vi "Get Next.vi"(7 "Q Ref In":refnum<queue>, 8 "error in":errorcluster) -> (0 "error out":errorcluster, 2 "Packet ID":string, 3 "Payload":variant, 5 "Q Ref Out":refnum<queue>)   [LabVIEW 2025, in "Q Wrappers.lvlib"]
uses:
  Q Wrappers.lvlib
  Q Packet.ctl
panel:
  in  "timeout (msec)":i32=-1
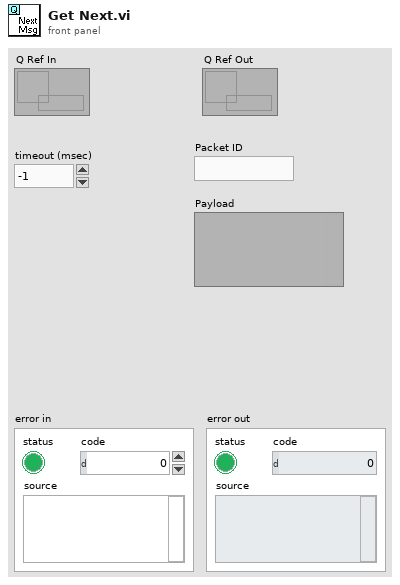
[diagram p1: front panel]
types:
  T1 = typedef "Q Packet.ctl" = cluster{"Packet ID":string, "Payload":variant}
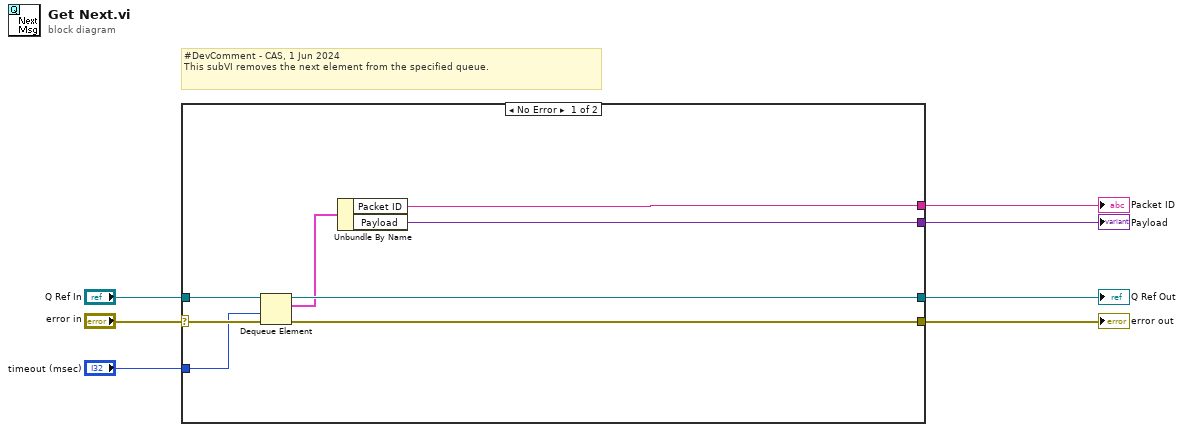
[diagram p0: block diagram]
diagram:
  # "#DevComment - CAS, 1 Jun 2024\nThis subVI removes the next element from the specified queue."
  n1 = case shown="No Error" "error in" {
    selector: "error in" -> [w15 w16]
    tunnel: [w14 w16] -> w6
    tunnel: [w13 _] -> w5
    tunnel: "Q Ref In" -> [w12 _]
    tunnel: [w10 _] -> w3
    tunnel: [w9 _] -> w2
    tunnel: "timeout (msec)" -> [w8 _]
    frame No Error {
      n2 = Dequeue Element(queue=w12, timeout in ms (-1)=w8, error in (no error)=w15) -> (queue out=w13:refnum<queue>, element=w11:T1, error out=w14:errorcluster)  [unwired: 1 out]
      n3 = Unbundle By Name(w11) -> ("Packet ID"=w10:string, "Payload"=w9:variant)
    }
    frame Error {
    }
  }
  "error out" <- w6
  "Q Ref Out" <- w5
  "Packet ID" <- w3
  "Payload" <- w2
